vi "Command with Logging.vi"(8 "error in":errorcluster, 10 "Event Details":T1, 11 "Instruments in":refnum<class "Instruments.lvclass">) -> (0 "error out":errorcluster, 3 "Instruments out":refnum<class "Instruments.lvclass">)   [LabVIEW 2023, in "Instruments.lvlib" / "Instruments.lvclass"]
uses:
  Library/Instruments.lvclass
  C:/Users/Public/Documents/Development/builds/Engine/Engine.lvlibp/Project/Engine.lvclass
  C:/Users/Public/Documents/Development/builds/Engine/Actor Framework.lvlibp/1abvi3w/vi.lib/ActorFramework/Actor/Actor.lvclass
  builds/Engine/Engine.lvlibp/Accessors/Read Report Queue.vi
  builds/Engine/Actor Framework.lvlibp/1abvi3w/vi.lib/ActorFramework/Actor/Read Actor Label.vi
  builds/Tools/QDMH.lvlibp/Private/Enqueue Bundled Element.vi
  builds/Tools/QDMH.lvlibp/QDMH.lvclass
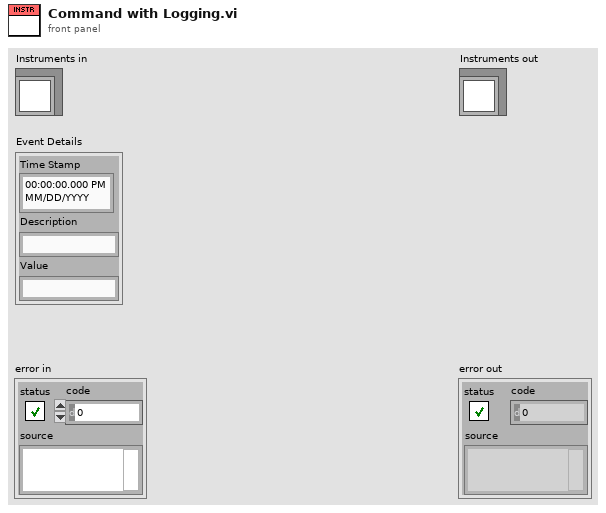
[diagram p1: front panel]
types:
  T1 = cluster{"Time Stamp":timestamp, "Description":string, "Value":string}
  T2 = cluster{"Time Stamp":timestamp, "Accessors:Actor Label":string, "Description":string, "Value":string}
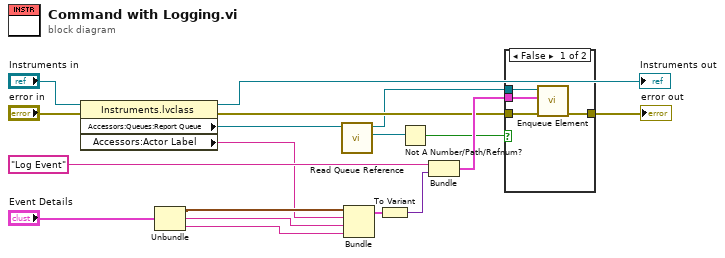
[diagram p0: block diagram]
diagram:
  n1 = property class="Instruments.lvclass"(reference="Instruments in", error in="error in") -> (reference out=→"Instruments out":refnum<class "Instruments.lvclass">, error out=w10:errorcluster, "Accessors:Queues:Report Queue"=w4:refnum<class "QDMH.lvclass">, "Accessors:Actor Label"=w7:string)
  n2 = Unbundle("Event Details") -> ("Time Stamp"=w8:timestamp, "Description"=w6:string, "Value"=w5:string)
  n3 = call "Read Queue Reference.vi"("QDMH in"=w4) -> ("Queue Reference"=w2:refnum<queue>, "QDMH out"=w3:refnum<class "QDMH.lvclass">)  [unwired: 8 in, 1 out]
  n4 = Bundle("Time Stamp"=w8, "Accessors:Actor Label"=w7, "Description"=w6, "Value"=w5) -> (w14:T2)  [unwired: 1 in]
  n5 = To Variant(anything=w14) -> (Variant=w13:variant)
  n6 = Not A Number/Path/Refnum?(number/path/refnum=w2) -> (NaN/Path/Refnum?=w1:bool)
  n7 = Bundle("Log Event", "Variant"=w13) -> (w12:cluster{string, "Variant":variant})  [unwired: 1 in]
  n8 = case shown="False" w1 {
    tunnel: [w22 w23] -> w18
    tunnel: w12 -> [w21 _]
    tunnel: w10 -> [w20 w23]
    tunnel: w3 -> [w19 _]
    frame False {
      n9 = call-poly "Enqueue Element.vi"("error in"=w20, "element"=w21, "QDMH in"=w19) -> ("error out"=w22:errorcluster)  [unwired: 7 in, 1 out]
    }
    frame True {
    }
  }
  "error out" <- w18
